vi "Add Method to Tree.vi"(0 "Message Maker in":refnum<class "Message Maker.lvclass">, 2 "Actor/Interface Refnum":refnum<vi>, 3 "Method VI Refnum":refnum<vi>, 5 "error in (no error)":errorcluster, 6 "Actor/Interface Tag":string) -> (14 "Message Maker out":refnum<class "Message Maker.lvclass">, 15 "Message Status":T1, 16 "Is Public Method":bool, 19 "error out":errorcluster)   [LabVIEW 2023, in "Message Maker.lvclass"]
uses:
  Message Maker.lvclass
  Message Status.ctl
  Message Maker.lvclass/Message Maker.ctl
panel:
  in  "Actor/Interface Tag 2":string
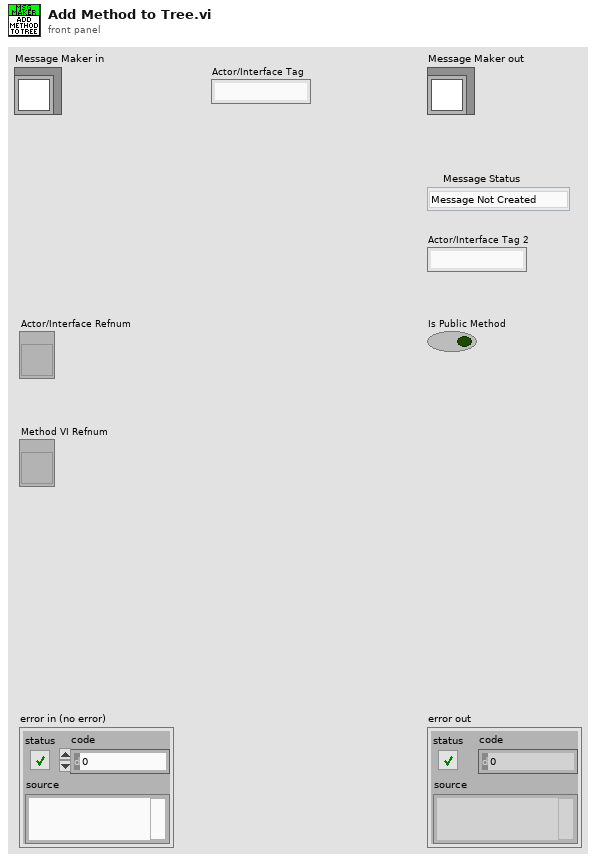
[diagram p1: front panel]
types:
  T1 = typedef "Message Maker.lvclass/Message Status.ctl" = enum16{"Message Not Created", "Message Out of Date", "Message OK", "Never update"}
  T2 = enum32{"invalid scope", "public", "private", "protected", "community"}
  T3 = enum32{"invalid VI type", "Standard VI", "Control VI", "Global VI", "Polymorphic VI", "Configuration VI", "SubSystem", "Facade VI", "Method VI", "Statechart Diagram VI"}
  T4 = typedef "Message Maker.lvclass/Details Map.ctl" = map{string, string}
  T5 = typedef "Message Maker.lvclass/Message Recipient Type.ctl" = enum16{"Actor", "Interface", "Async Actor"}
  T6 = typedef "Message Maker.lvclass/Message Type.ctl" = enum16{"Standard", "Async"}
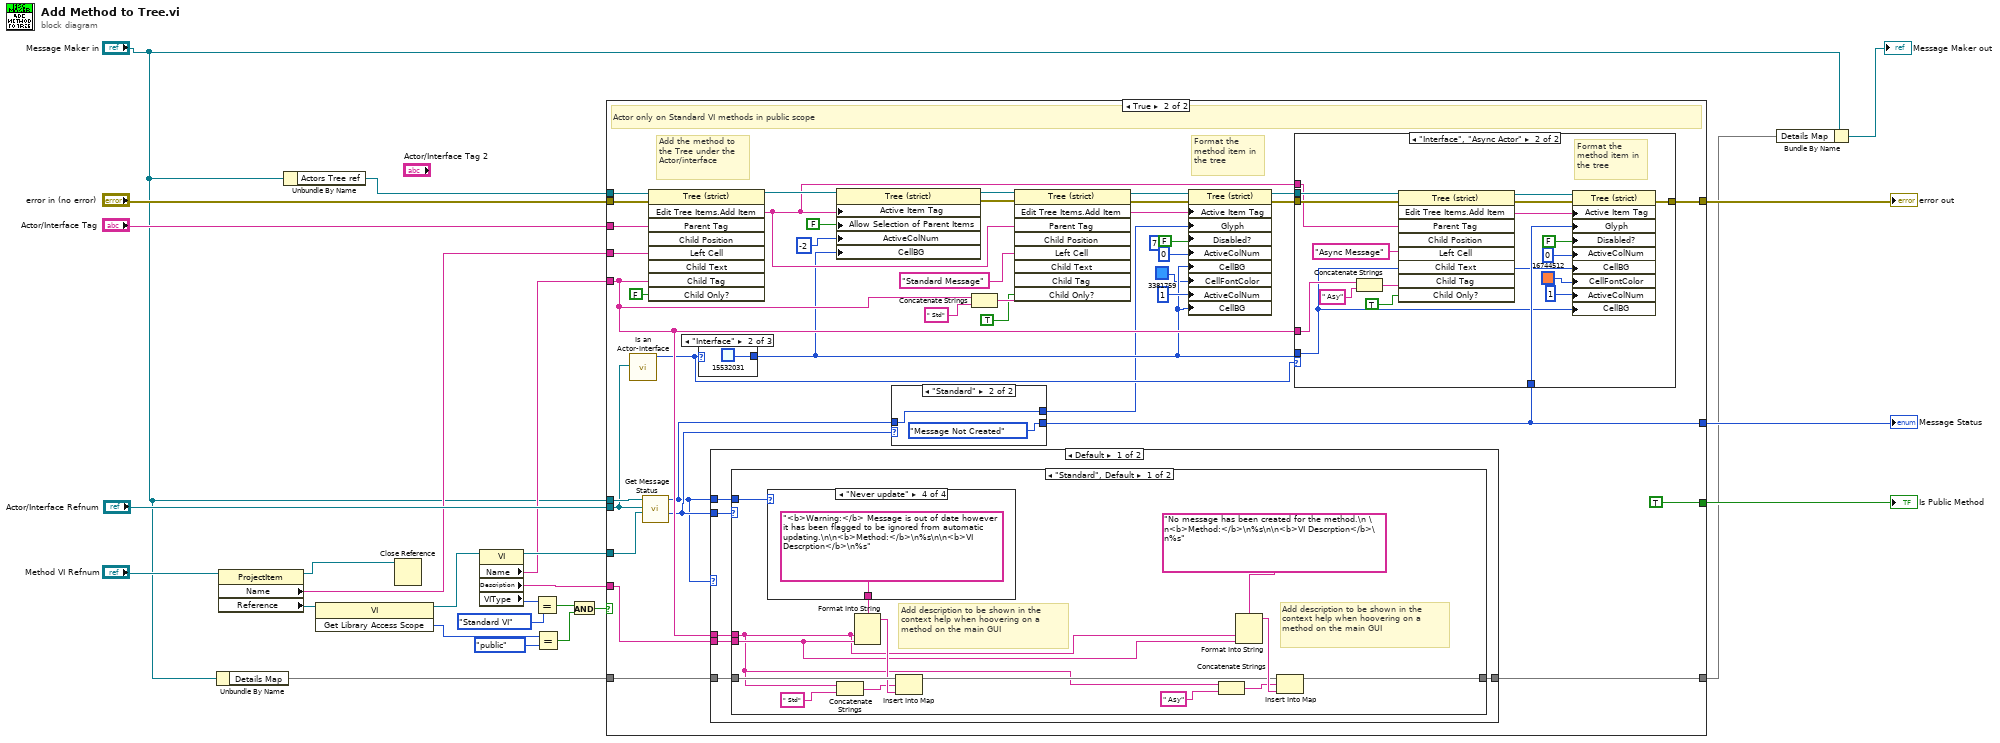
[diagram p0: block diagram]
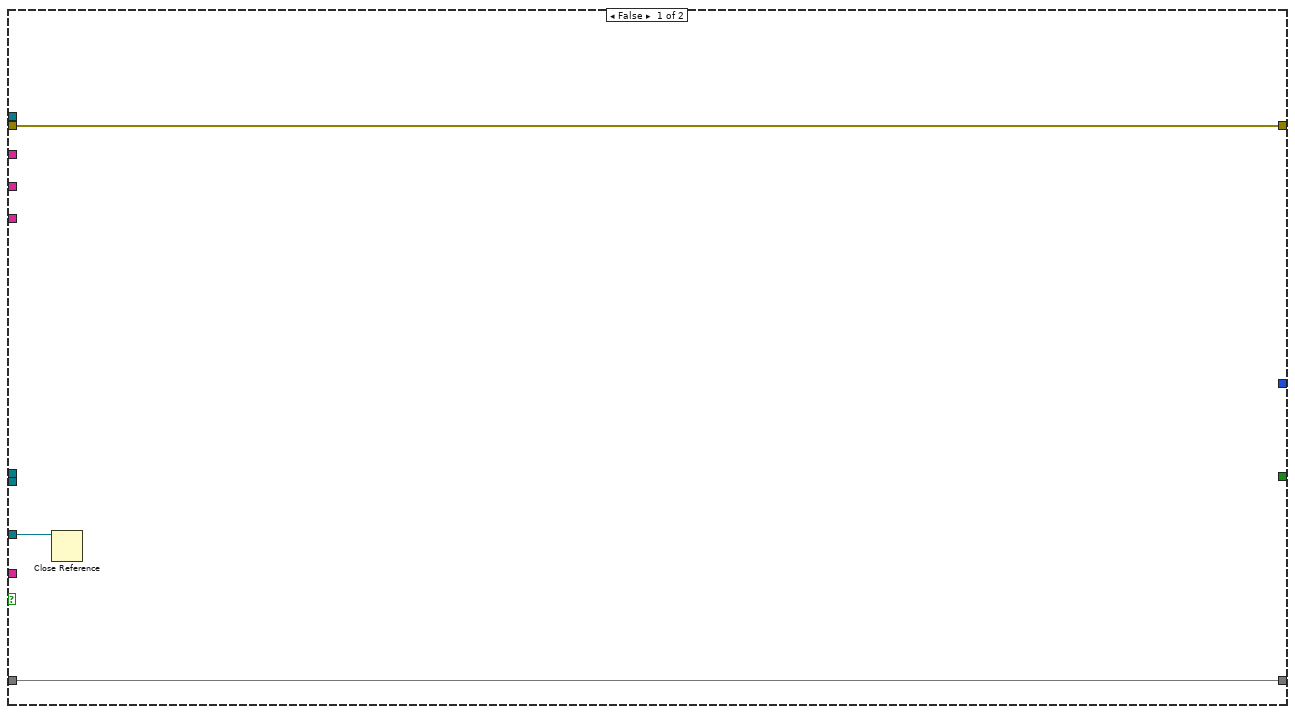
[diagram p2: hidden frame]
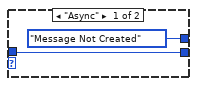
[diagram p3: hidden frame]
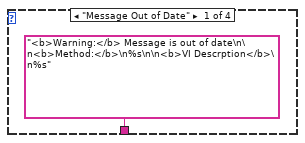
[diagram p4: hidden frame]
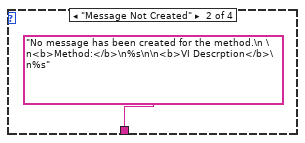
[diagram p5: hidden frame]
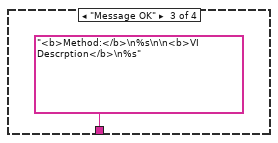
[diagram p6: hidden frame]
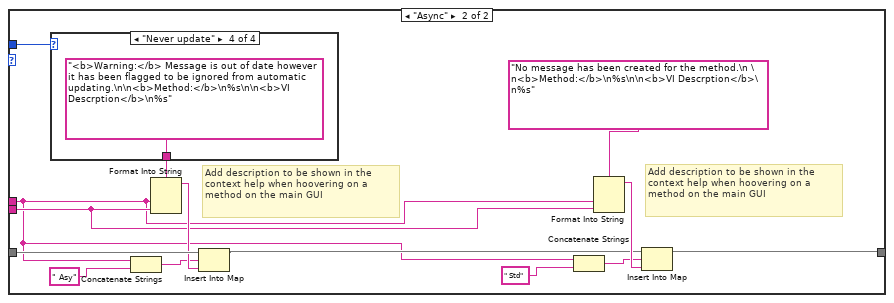
[diagram p7: hidden frame]
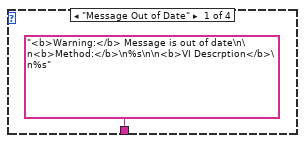
[diagram p8: hidden frame]
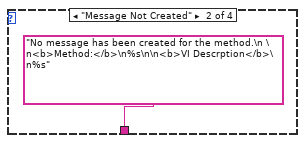
[diagram p9: hidden frame]
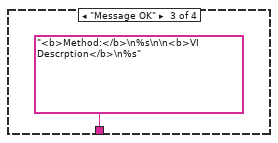
[diagram p10: hidden frame]
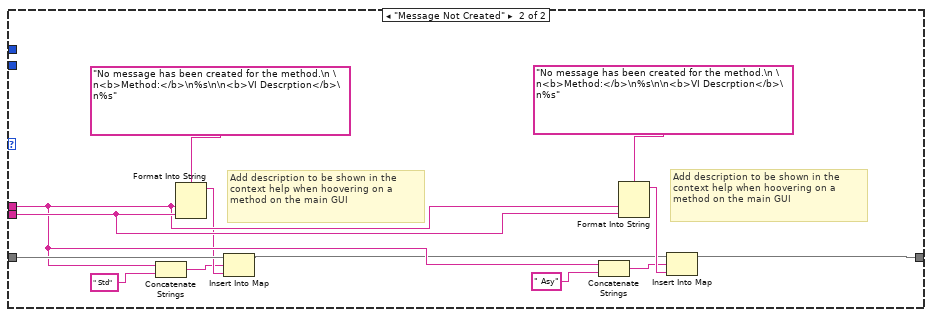
[diagram p11: hidden frame]
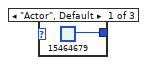
[diagram p12: hidden frame]
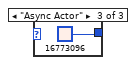
[diagram p13: hidden frame]
diagram:
  n1 = Unbundle By Name("Message Maker in") -> ("Details Map"=w4:T4)
  n2 = property class="ProjectItem"(reference="Method VI Refnum") -> (reference out=w9:refnum<vi>, "Name"=w7:string, "Reference"=w11:refnum<vi>)  [unwired: 1 in, 1 out]
  n3 = Unbundle By Name("Message Maker in") -> ("Actors Tree ref"=w5:refnum<vi>)
  n4 = invoke class="VI" method="Get Library Access Scope"(reference=w11) -> (reference out=w14:refnum<vi>, "Get Library Access Scope"=w19:T2)  [unwired: 2 in, 1 out]
  n5 = Close Reference(reference=w9) -> ()  [unwired: 1 in, 1 out]
  n6 = property class="VI"(reference=w14) -> (reference out=w22:refnum<vi>, "Name"=w12:string, "Description"=w13:string, "VIType"=w15:T3)  [unwired: 1 in, 1 out]
  n7 = Equal?(x=w15, y=T3."Standard VI") -> (x = y?=w16:bool)
  n8 = Equal?(x=w19, y=T2."public") -> (x = y?=w18:bool)
  n9 = And(x=w16, y=w18) -> (x .and. y?=w21:bool)
  n10 = case shown="True" w21 {
    tunnel: w5 -> [_ w68]
    tunnel: "error in (no error)" -> [w29 w67]
    tunnel: w7 -> [_ w66]
    tunnel: "Actor/Interface Tag" -> [_ w65]
    tunnel: [w29 w43] -> w10
    tunnel: w12 -> [_ w41]
    tunnel: w13 -> [_ w46]
    tunnel: [w28 w40] -> w3
    tunnel: w4 -> [w28 w63]
    tunnel: w22 -> [w27 w48]
    tunnel: "Actor/Interface Refnum" -> [_ w37]
    tunnel: [_ w31] -> w24
    tunnel: [_ TRUE] -> w25
    tunnel: "Message Maker in" -> [_ w47]
    frame False {
      n11 = Close Reference(reference=w27) -> ()  [unwired: 1 in, 1 out]
    }
    frame True {
      (unwired) 7 ("Active Item:Symbol Index")
      # "Format the method item in the tree"
      # "Add the method to the Tree under the Actor/interface"
      # "Actor only on Standard VI methods in public scope"
      n12 = call "Is an Actor-Interface.vi"("Class in"=w37) -> ("Message Recipient Type"=w36:T5)  [unwired: 14 in, 4 out]
      n13 = call "Get Message Status.vi"("VI"=w48, "Actor Class"=w37, "Message Maker in"=w47) -> ("Message Type"=w33:T6, "Message Status"=w32:T1)  [unwired: 7 in]
      n14 = invoke class="Tree (strict)" method="Edit Tree Items.Add Item"(reference=w68, error in=w67, "Parent Tag"=w65, "Left Cell"=w66, "Child Tag"=w41, "Child Only?"=FALSE) -> (reference out=w52:refnum<vi>, "Edit Tree Items:Add Item"=w42:string)  [unwired: 3 in, 7 out]
      n15 = case shown="\"Interface\"" w36 {
        tunnel: [u32 15464679 u32 15532031 u32 16773096] -> w35
        frame "Actor", Default {
        }
        frame "Interface" {
        }
        frame "Async Actor" {
        }
      }
      n16 = case shown="Default" w32 {
        tunnel: w63 -> [w78 w127]
        tunnel: w46 -> [w77 w126]
        tunnel: w41 -> [w76 w125]
        tunnel: [w75 w124] -> w40
        tunnel: w32 -> [w74 _]
        tunnel: w33 -> [w73 _]
        frame Default {
          n17 = case shown="\"Standard\", Default" w73 {
            tunnel: w78 -> [w92 w110]
            tunnel: w77 -> [w82 w102]
            tunnel: w76 -> [w80 w100]
            tunnel: [w79 w97] -> w75
            tunnel: w74 -> [w87 w106]
            frame "Standard", Default {
              # "Add description to be shown in the context help when hoovering on a method on the main GUI"
              # "Add description to be shown in the context help when hoovering on a method on the main GUI"
              n18 = case shown="\"Never update\"" w87 {
                tunnel: ["<b>Warning:</b> Message is out of date\n\n<b>Method:</b>\n%s\n\n<b>VI Descrption</b>\n%s" ("format string") "No message has been created for the method.\n \n<b>Method:</b>\n%s\n\n<b>VI Descrption</b>\n%s" ("format string") "<b>Method:</b>\n%s\n\n<b>VI Descrption</b>\n%s" ("format string") "<b>Warning:</b> Message is out of date however it has been flagged to be ignored from automatic updating.\n\n<b>Method:</b>\n%s\n\n<b>VI Descrption</b>\n%s" ("format string")] -> w91
                frame "Message Out of Date" {
                }
                frame "Message Not Created" {
                }
                frame "Message OK" {
                }
                frame "Never update" {
                }
              }
              n19 = Concatenate Strings(w80, " Std" ("string")) -> (w89:string)
              n20 = Format Into String(format string=w91, w80, w82) -> (resulting string=w90:string)  [unwired: 2 in, 1 out]
              n21 = Insert Into Map(map in=w92, key=w89, value=w90) -> (map out=w81:T4)  [unwired: 2 out]
              n22 = Concatenate Strings(w80, " Asy" ("string")) -> (w84:string)
              n23 = Format Into String(format string="No message has been created for the method.\n \n<b>Method:</b>\n%s\n\n<b>VI Descrption</b>\n%s", w80, w82) -> (resulting string=w85:string)  [unwired: 2 in, 1 out]
              n24 = Insert Into Map(map in=w81, key=w84, value=w85) -> (map out=w79:T4)  [unwired: 2 out]
            }
            frame "Async" {
              # "Add description to be shown in the context help when hoovering on a method on the main GUI"
              # "Add description to be shown in the context help when hoovering on a method on the main GUI"
              n25 = case shown="\"Never update\"" w106 {
                tunnel: ["<b>Warning:</b> Message is out of date\n\n<b>Method:</b>\n%s\n\n<b>VI Descrption</b>\n%s" ("format string") "No message has been created for the method.\n \n<b>Method:</b>\n%s\n\n<b>VI Descrption</b>\n%s" ("format string") "<b>Method:</b>\n%s\n\n<b>VI Descrption</b>\n%s" ("format string") "<b>Warning:</b> Message is out of date however it has been flagged to be ignored from automatic updating.\n\n<b>Method:</b>\n%s\n\n<b>VI Descrption</b>\n%s" ("format string")] -> w109
                frame "Message Out of Date" {
                }
                frame "Message Not Created" {
                }
                frame "Message OK" {
                }
                frame "Never update" {
                }
              }
              n26 = Concatenate Strings(w100, " Asy" ("string")) -> (w107:string)
              n27 = Format Into String(format string=w109, w100, w102) -> (resulting string=w108:string)  [unwired: 2 in, 1 out]
              n28 = Insert Into Map(map in=w110, key=w107, value=w108) -> (map out=w101:T4)  [unwired: 2 out]
              n29 = Concatenate Strings(w100, " Std" ("string")) -> (w103:string)
              n30 = Format Into String(format string="No message has been created for the method.\n \n<b>Method:</b>\n%s\n\n<b>VI Descrption</b>\n%s", w100, w102) -> (resulting string=w104:string)  [unwired: 2 in, 1 out]
              n31 = Insert Into Map(map in=w101, key=w103, value=w104) -> (map out=w97:T4)  [unwired: 2 out]
            }
          }
        }
        frame "Message Not Created" {
          # "Add description to be shown in the context help when hoovering on a method on the main GUI"
          # "Add description to be shown in the context help when hoovering on a method on the main GUI"
          n32 = Concatenate Strings(w125, " Std" ("string")) -> (w121:string)
          n33 = Format Into String(format string="No message has been created for the method.\n \n<b>Method:</b>\n%s\n\n<b>VI Descrption</b>\n%s", w125, w126) -> (resulting string=w122:string)  [unwired: 2 in, 1 out]
          n34 = Insert Into Map(map in=w127, key=w121, value=w122) -> (map out=w115:T4)  [unwired: 2 out]
          n35 = Concatenate Strings(w125, " Asy" ("string")) -> (w117:string)
          n36 = Format Into String(format string="No message has been created for the method.\n \n<b>Method:</b>\n%s\n\n<b>VI Descrption</b>\n%s", w125, w126) -> (resulting string=w118:string)  [unwired: 2 in, 1 out]
          n37 = Insert Into Map(map in=w115, key=w117, value=w118) -> (map out=w124:T4)  [unwired: 2 out]
        }
      }
      n38 = property class="Tree (strict)"(reference=w52, "Active Item Tag"=w42, "Allow Selection of Parent Items"=FALSE ("Expand/Contract Symbol:Show Symbol at Root"), "ActiveColNum"=-2 ("Active Cell:Active Column Number"), "CellBG"=w35) -> (reference out=w50:refnum<vi>, error out=w49:errorcluster)  [unwired: 1 in]
      n39 = case shown="\"Standard\"" w33 {
        tunnel: w32 -> [w70 w71]
        tunnel: [w70 Message_Status."Message Not Created" ("Message Status")] -> w31
        tunnel: [Message_Status."Message Not Created" ("Message Status") w71] -> w30
        frame "Async" {
        }
        frame "Standard" {
        }
      }
      n40 = Concatenate Strings(w41, " Std" ("string")) -> (w55:string)
      n41 = invoke class="Tree (strict)" method="Edit Tree Items.Add Item"(reference=w50, error in=w49, "Parent Tag"=w42, "Left Cell"="Standard Message" ("Left Cell String"), "Child Tag"=w55, "Child Only?"=TRUE) -> (reference out=w58:refnum<vi>, error out=w59:errorcluster, "Edit Tree Items:Add Item"=w56:string)  [unwired: 3 in, 6 out]
      n42 = property on="Property Node" class="Tree (strict)"(reference=w58, error in=w59, "Active Item Tag"=w56, "Glyph"=w30, "Disabled?"=FALSE ("Active Item:Disabled?"), "ActiveColNum"=0 ("Active Cell:Active Column Number"), "CellBG"=w35, "CellFontColor"=u32 3381759 ("Active Cell:Cell Font:Color"), "ActiveColNum"=1 ("Active Cell:Active Column Number"), "CellBG"=w35) -> (reference out=w45:refnum<vi>, error out=w44:errorcluster)
      n43 = case shown="\"Interface\", \"Async Actor\"" w36 {
        tunnel: w45 -> [_ w140]
        tunnel: w44 -> [w131 w139]
        tunnel: [w131 w138] -> w43
        tunnel: w31 -> [_ w137]
        tunnel: w42 -> [_ w136]
        tunnel: w41 -> [_ w135]
        tunnel: w35 -> [_ w133]
        frame "Actor", Default {
        }
        frame "Interface", "Async Actor" {
          # "Format the method item in the tree"
          n44 = Concatenate Strings(w135, " Asy" ("string")) -> (w149:string)
          n45 = invoke class="Tree (strict)" method="Edit Tree Items.Add Item"(reference=w140, error in=w139, "Parent Tag"=w136, "Left Cell"="Async Message" ("Left Cell String"), "Child Tag"=w149, "Child Only?"=TRUE) -> (reference out=w147:refnum<vi>, error out=w146:errorcluster, "Edit Tree Items:Add Item"=w148:string)  [unwired: 3 in, 6 out]
          n46 = property on="Property Node" class="Tree (strict)"(reference=w147, error in=w146, "Active Item Tag"=w148, "Glyph"=w137, "Disabled?"=FALSE ("Active Item:Disabled?"), "ActiveColNum"=0 ("Active Cell:Active Column Number"), "CellBG"=w133, "CellFontColor"=u32 16744512 ("Active Cell:Cell Font:Color"), "ActiveColNum"=1 ("Active Cell:Active Column Number"), "CellBG"=w133) -> (error out=w138:errorcluster)  [unwired: 1 out]
        }
      }
    }
  }
  "Is Public Method" <- w25
  "Message Status" <- w24
  "error out" <- w10
  n47 = Bundle By Name(cluster="Message Maker in", "Details Map"=w3) -> (→"Message Maker out":refnum<class "Message Maker.lvclass">)
